vi "DMM_Verify Instrument Options - Versions.vi"(8 "error in (no error)":errorcluster, 11 "PXIe-4071 in":refnum<class "PXIe-4071.lvclass">) -> (0 "error out":errorcluster, 3 "PXIe-4071 out":refnum<class "PXIe-4071.lvclass">)   [LabVIEW 2018, in "PXIe-4071.lvclass"]
uses:
  PXIe-4071.lvclass
  Controls/Instrument Attributes Cluster.ctl
  PXIe-4071.lvclass/PXIe-4071.ctl
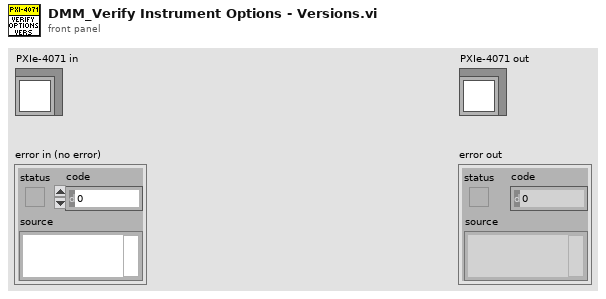
[diagram p1: front panel]
types:
  T1 = typedef "Instrument Attributes Cluster.ctl" = cluster{"Reported Firmware Rev":string, "Reported Options":string}
  T2 = typedef "Class Instrument Info.ctl" = string[]
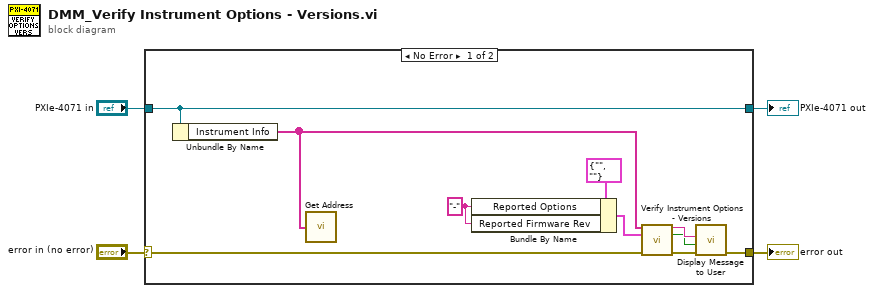
[diagram p0: block diagram]
diagram:
  n1 = case shown="No Error" "error in (no error)" {
    selector: "error in (no error)" -> [w6 w16]
    tunnel: [w11 w16] -> w4
    tunnel: [w10 w15] -> w2
    tunnel: "PXIe-4071 in" -> [w10 w15]
    frame No Error {
      w5 = "-" ("Reported Options")
      n2 = Unbundle By Name(w10) -> ("Instrument Info"=w7:T2)
      n3 = call "Get Address.vi"("Instrument Info"=w7) -> ()  [unwired: 4 in, 1 out]
      n4 = Bundle By Name(cluster=T1 {"Reported Firmware Rev"="", "Reported Options"=""} ("Instrument Attributes"), "Reported Options"=w5, "Reported Firmware Rev"=w5) -> (w8:T1)
      n5 = call "Verify Instrument Options - Versions.vi"("Instrument Info"=w7, "Instrument Attributes"=w8, "error in (no error)"=w6) -> ("Options & Versions Validation"=w14:string, "Mismatch? (True = Mismatch)"=w13:bool, "error out"=w12:errorcluster)  [unwired: 10 in]
      n6 = call "Display Message to User"("error in (no error)"=w12, "Enable"=w13, "Message"=w14) -> ("error out"=w11:errorcluster)  [unwired: 7 in, 1 out]
    }
    frame Error {
    }
  }
  "PXIe-4071 out" <- w2
  "error out" <- w4
